vi "build_T1_curve-2017.07.24.vi"(8 "T1_parameters":T1, 9 "timetags":u32[][](array[numeric]), 10 "stop_read":u32[][](array[numeric]), 11 "start_read":u32[][](array[numeric])) -> (2 "T1 curve":cluster{dbl[], "dark_time_us":dbl[]}, 3 "std_measures":dbl[](array[numeric]))   [LabVIEW 2014]
uses:
  <vilib>/Analysis/NI_AALBase.lvlib
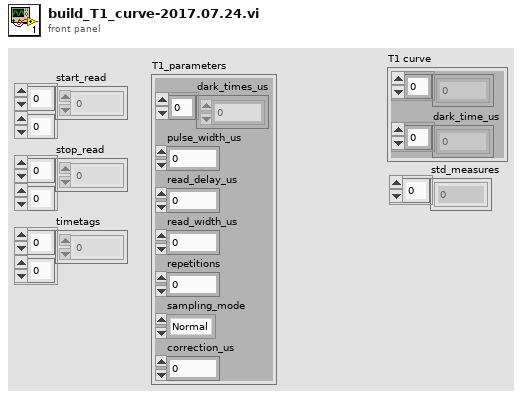
[diagram p1: front panel]
types:
  T1 = cluster{"dark_times_us":dbl[], "pulse_width_us":dbl, "read_delay_us":dbl, "read_width_us":dbl, "repetitions":i32, "sampling_mode":enum16{"Normal", "Sweep"}, "correction_us":dbl}
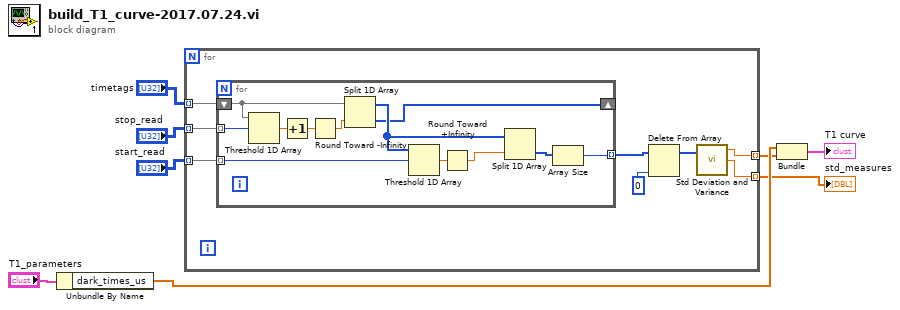
[diagram p0: block diagram]
diagram:
  n1 = Unbundle By Name("T1_parameters") -> ("dark_times_us"=w6:dbl[])
  n2 = for {
    tunnel: "timetags" -> [w16] mode=indexing
    tunnel: [w12] -> w5 mode=indexing
    tunnel: [w11] -> w4 mode=indexing
    tunnel: "start_read" -> [w10] mode=indexing
    tunnel: "stop_read" -> [w9] mode=indexing
    n3 = for {
      tunnel: w10 -> [w21] mode=indexing
      tunnel: w9 -> [w28] mode=indexing
      shift-right: [w23] -> _
      shift-left: w16 -> [w24]
      tunnel: [w22] -> w14 mode=indexing
      n4 = Threshold 1D Array(2:w28, 3:w24) -> (0:w25:dbl)  [unwired: 1 in]
      n5 = Increment(x=w25) -> (x+1=w20:dbl)
      n6 = Round Toward -Infinity(1:w20) -> (0:w17:dbl)
      n7 = Split 1D Array(array=w24, index=w17) -> (first subarray=w26:u32[], second subarray=w23:u32[])
      n8 = Threshold 1D Array(2:w21, 3:w26) -> (0:w27:dbl)  [unwired: 1 in]
      n9 = Round Toward +Infinity(x=w27) -> (ceil(x): smallest int >= x=w19:dbl)
      n10 = Split 1D Array(array=w26, index=w19) -> (second subarray=w18:u32[])  [unwired: 1 out]
      n11 = Array Size(array=w18) -> (size(s)=w22:i32)
    }
    n12 = Delete From Array(array=w14, index=0) -> (array with subset deleted=w13:i32[])  [unwired: 1 in, 1 out]
    n13 = call <vilib>:"Std Deviation and Variance.vi"("X"=w13) -> ("mean"=w12:dbl, "standard deviation"=w11:dbl)  [unwired: 1 in, 1 out]
  }
  "std_measures" <- w4
  n14 = Bundle("dark_times_us"=w6, w5) -> (→"T1 curve":cluster{"dark_times_us":dbl[], dbl[]})  [unwired: 1 in]
